vi "LSX Get Calibrate Dir.vi"(0 "lLSID":i32, 1 "plAD":i32, 5 "plXD":i32, 7 "plYD":i32, 9 "plZD":i32, 11 "error in (no error)":errorcluster) -> (3 "plAD out":i32, 4 "function return":i32, 6 "plXD out":i32, 8 "plYD out":i32, 10 "plZD out":i32, 15 "error out":errorcluster)   [LabVIEW 2018, in "Tango.lvlib"]
doc: "TANGOAPI int TANGOCALL LSX_GetCalibrateDir (int lLSID, int *plXD, int *plYD, int *plZD, int *plAD);"
uses:
  <userlib>/Tango/Tango.lvlib
  <userlib>/Tango/Tango_DLL.dll
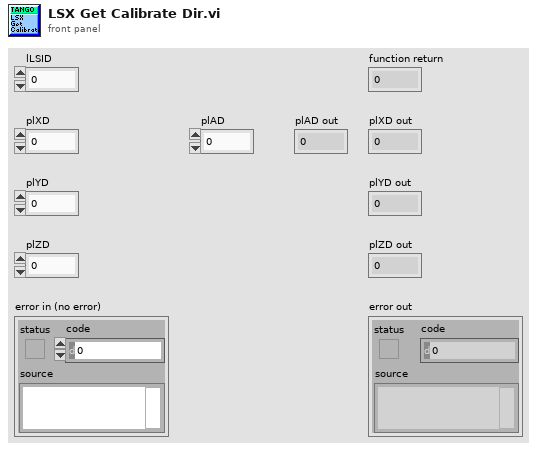
[diagram p1: front panel]
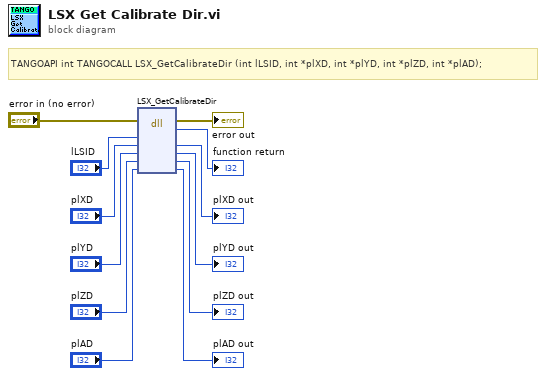
[diagram p0: block diagram]
diagram:
  # "TANGOAPI int TANGOCALL LSX_GetCalibrateDir (int lLSID, int *plXD, int *plYD, int *plZD, int *plAD);"
  n1 = dll-call lib="C:/Program Files (x86)/National Instruments/LabVIEW 2018/user.lib/Tango/Tango_DLL.*" fn="LSX_GetCalibrateDir"(error in="error in (no error)", "lLSID"="lLSID", "plXD"="plXD", "plYD"="plYD", "plZD"="plZD", "plAD"="plAD") -> (error out=→"error out":errorcluster, →"function return":i32, "plXD"=→"plXD out":i32, "plYD"=→"plYD out":i32, "plZD"=→"plZD out":i32, "plAD"=→"plAD out":i32)  [unwired: 3 in, 1 out]
